vi "Get LocalPath.vi"(8 "error in (no error)":errorcluster, 11 "FileTransfer in":refnum<class "FileTransfer.lvclass">) -> (0 "error out":errorcluster, 2 "LocalPath":string, 3 "FileTransfer out":refnum<class "FileTransfer.lvclass">)   [LabVIEW 2015, in "WinSCP.lvlib" / "FileTransfer.lvclass"]
uses:
  FileTransfer.lvclass
  FileTransfer.lvclass/FileTransfer.ctl
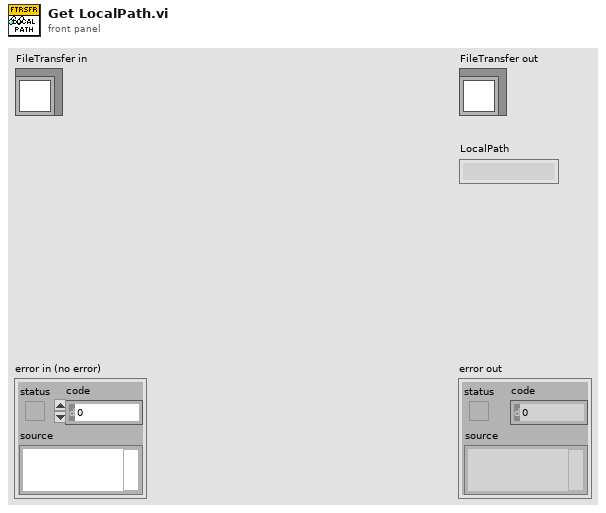
[diagram p1: front panel]
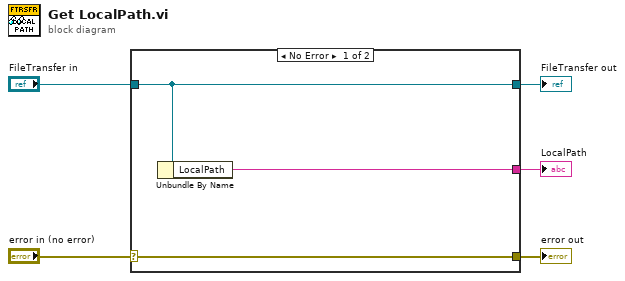
[diagram p0: block diagram]
diagram:
  n1 = case shown="No Error" "error in (no error)" {
    selector: "error in (no error)" -> [w8 w9]
    tunnel: [w8 w9] -> w4
    tunnel: [w7 w10] -> w2
    tunnel: "FileTransfer in" -> [w7 w10]
    tunnel: [w6 _] -> w1
    frame No Error {
      n2 = Unbundle By Name(w7) -> ("LocalPath"=w6:string)
    }
    frame Error {
    }
  }
  "error out" <- w4
  "FileTransfer out" <- w2
  "LocalPath" <- w1
